vi "All Library Descendants.vi"(8 "error in (no error)":errorcluster, 11 "Library in":refnum<vi>) -> (0 "error out":errorcluster, 1 "VIs":refnum<vi>[](array[refnum]), 2 "Libraries":refnum<vi>[](array[refnum]), 3 "Library":refnum<vi>)   [LabVIEW 2020, in "LV-Protoc.lvlib"]
uses:
  LV-Protoc.lvlib
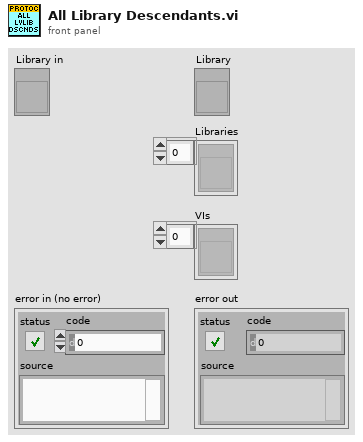
[diagram p1: front panel]
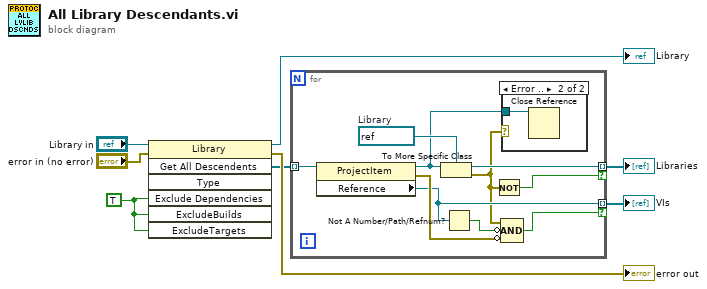
[diagram p0: block diagram]
diagram:
  w6 = TRUE ("ExcludeDependencies")
  n1 = invoke class="Library" method="Get All Descendents"(reference="Library in", error in="error in (no error)", "Exclude Dependencies"=w6, "ExcludeBuilds"=w6, "ExcludeTargets"=w6) -> (reference out=→"Library":refnum<vi>, error out=→"error out":errorcluster, "All Descendents"=w5:refnum<vi>[])  [unwired: 2 in, 4 out]
  n2 = for {
    tunnel: w5 -> [w18] mode=indexing
    tunnel: [w16] -> w4 mode=indexing if=w15
    tunnel: [w13] -> w3 mode=indexing if=w11
    w17 = refnum<vi> refnum  # Library
    n3 = property class="ProjectItem"(reference=w18) -> (reference out=w10:refnum<vi>, error out=w14:errorcluster, "Reference"=w13:refnum<vi>)  [unwired: 1 in]
    n4 = To More Specific Class(target class=w17, reference=w10) -> (specific class reference=w16:refnum<vi>, error out=w9:errorcluster)  [unwired: 1 in]
    n5 = Not A Number/Path/Refnum?(number/path/refnum=w13) -> (NaN/Path/Refnum?=w12:bool)
    n6 = Not(x=w9) -> (.not. x?=w15:bool)
    n7 = Compound Arithmetic op=AND(w9, invert w12, invert w14) -> (w11:bool)
    n8 = case shown="Error .." w9 {
      tunnel: w10 -> [_ w19]
      frame No Error {
      }
      frame Error {
        n9 = Close Reference(reference=w19) -> ()  [unwired: 1 in, 1 out]
      }
    }
  }
  "Libraries" <- w4
  "VIs" <- w3
